vi "Write Event Name and Time to Server.vi"(7 "Timer Value (ms)":dbl, 8 "error in (no error)":errorcluster, 9 "eventInfo":dbl=nan, 10 "Event Name":string, 11 "connection ID":refnum<k5>) -> (0 "error out":errorcluster, 3 "connection ID duplicate":refnum<k5>)   [LabVIEW 2014, in "Core SubVIs.lvlib"]
uses:
  Core SubVIs.lvlib
  Matlab API/Matlab API.lvlib
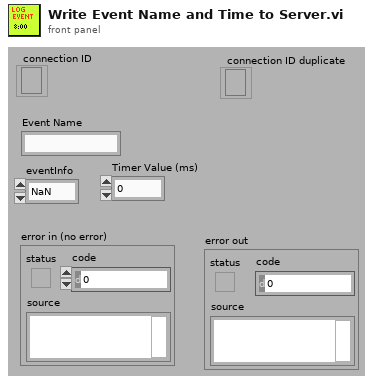
[diagram p1: front panel]
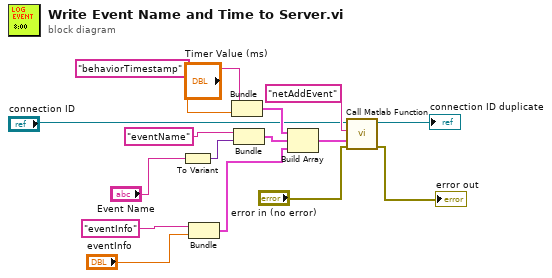
[diagram p0: block diagram]
diagram:
  n1 = To Variant(anything="Event Name") -> (Variant=w12:variant)
  n2 = Bundle("eventInfo", "eventInfo"="eventInfo") -> (w4:cluster{string, "eventInfo":dbl})  [unwired: 1 out]
  n3 = Bundle("behaviorTimestamp", "Timer Value (ms)"="Timer Value (ms)") -> (w14:cluster{string, "Timer Value (ms)":dbl})  [unwired: 1 out]
  n4 = Bundle("eventName", "Variant"=w12) -> (w13:cluster{string, "Variant":variant})  [unwired: 1 out]
  n5 = Build Array(w14, w13, w4) -> (w11:cluster{string, "Variant":variant}[])
  n6 = call "Call Matlab Function.vi"("error in (no error)"="error in (no error)", "Matlab Param Array"=w11, "Function name"="netAddEvent", "TCP Network Connection Refnum"="connection ID") -> ("error out"=→"error out":errorcluster, "connection ID out"=→"connection ID duplicate":refnum<k5>)  [unwired: 6 out]
